vi "main_TC.vi"() -> ()   [LabVIEW 2017]
uses:
  <vilib>/addons/control/pid/pid.llb/PID (DBL).vi
  <vilib>/addons/control/pid/NI_PID_pid.lvlib
panel:
  out "Control_OnToOff":bool
  out "Abs Control Action":dbl
  in  "Tab Control":enum32{"Page 1", "Page 2"}(tab)
  in  "ON/OFF":bool
  in  "PID gains":cluster{"Kp":dbl, "KI":dbl, "Kd":dbl}={"Kp"=1.0, "KI"=0.0, "Kd"=0.0}
  in  "Pause Button":bool
  in  "Reset Chart":bool
  in  "Save as Excel":bool
  in  "Save as image":bool
  in  "Block Diagram":bool
  out "T3":dbl
  out "T2":dbl
  out "T1":dbl
  out "Cooler":bool
  out "Heater":bool
  out "Actuator Used":enum16{"heater", "cooler", "None"}(ring)
  out "Control Action":dbl
  in  "Temperature setpoint":dbl=25.0
  in  "Actuator":bool=TRUE
  in  "ON/OFF Control Loop":bool caption="ON/OFF control loop"
  in  "Exit":bool
  out "NI1":tag caption="NI device"
  out "Waveform Chart":T1(graph) caption="Response Chart"
  in  "Main board":bool
  # "Temperature Control Training System"
  # "Sensors Reading"
  # "Block Diagram of \nthe Temperature Closed-loop Control System"
  # "1"
  # "3"
  # "ON/OFF"
  # "ON/OFF Control Loop"
  # "Actuator ON/OFF"
  # "2"
  # "Heat Genration or \nAbsorption"
  # "Controller\n(PID)"
  # "Actuator\n(Heater/Cooler)"
  # "desired   T"
  # "Rod"
  # "error signal"
  # "+"
  # "-"
  # "Control Action\n(-100% - 100%)"
  # "T1"
  # "Sensors"
  # "T2"
  # "T3"
  # "Operation Steps :"
  # "1) Turn the Trainer switch ON\n2) Set the desired temperature \n3)Turn On the Control Loop switch\n\nNote: You can reset the desired temperature \n           while the control loop is running."
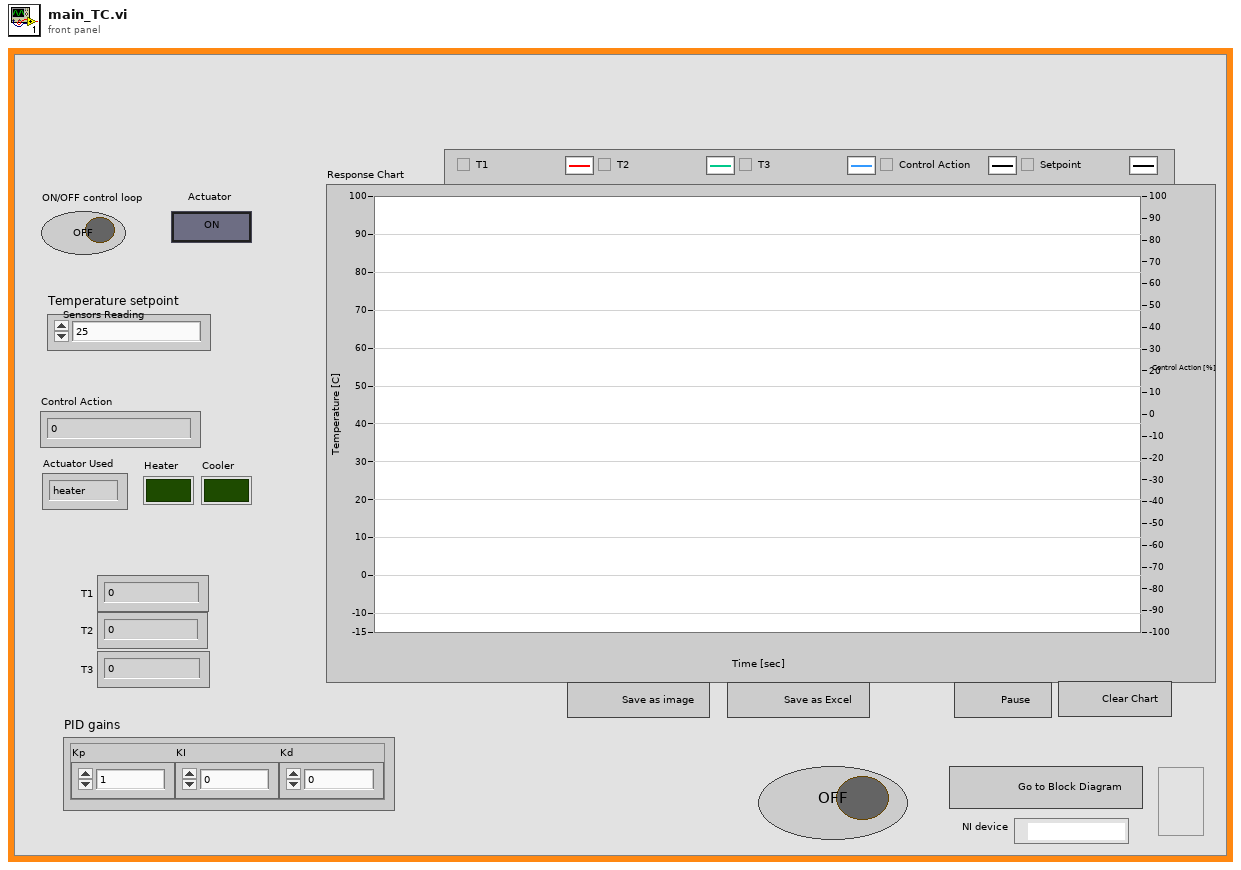
[diagram p1: front panel]
types:
  T1 = cluster{"Scalar":dbl, "Scalar":dbl, "Scalar":dbl, "f":dbl, "Temperature setpoint":dbl}
  T2 = enum32{"Invalid", "Standard", "Closed", "Hidden", "Minimized", "Maximized"}
  T3 = enum8{"Enabled", "Disabled", "Disabled and Grayed Out"}
  T4 = cluster{"Scalar":dbl, "Scalar":dbl, "Scalar":dbl, "f":dbl, "Temperature setpoint":dbl}[]
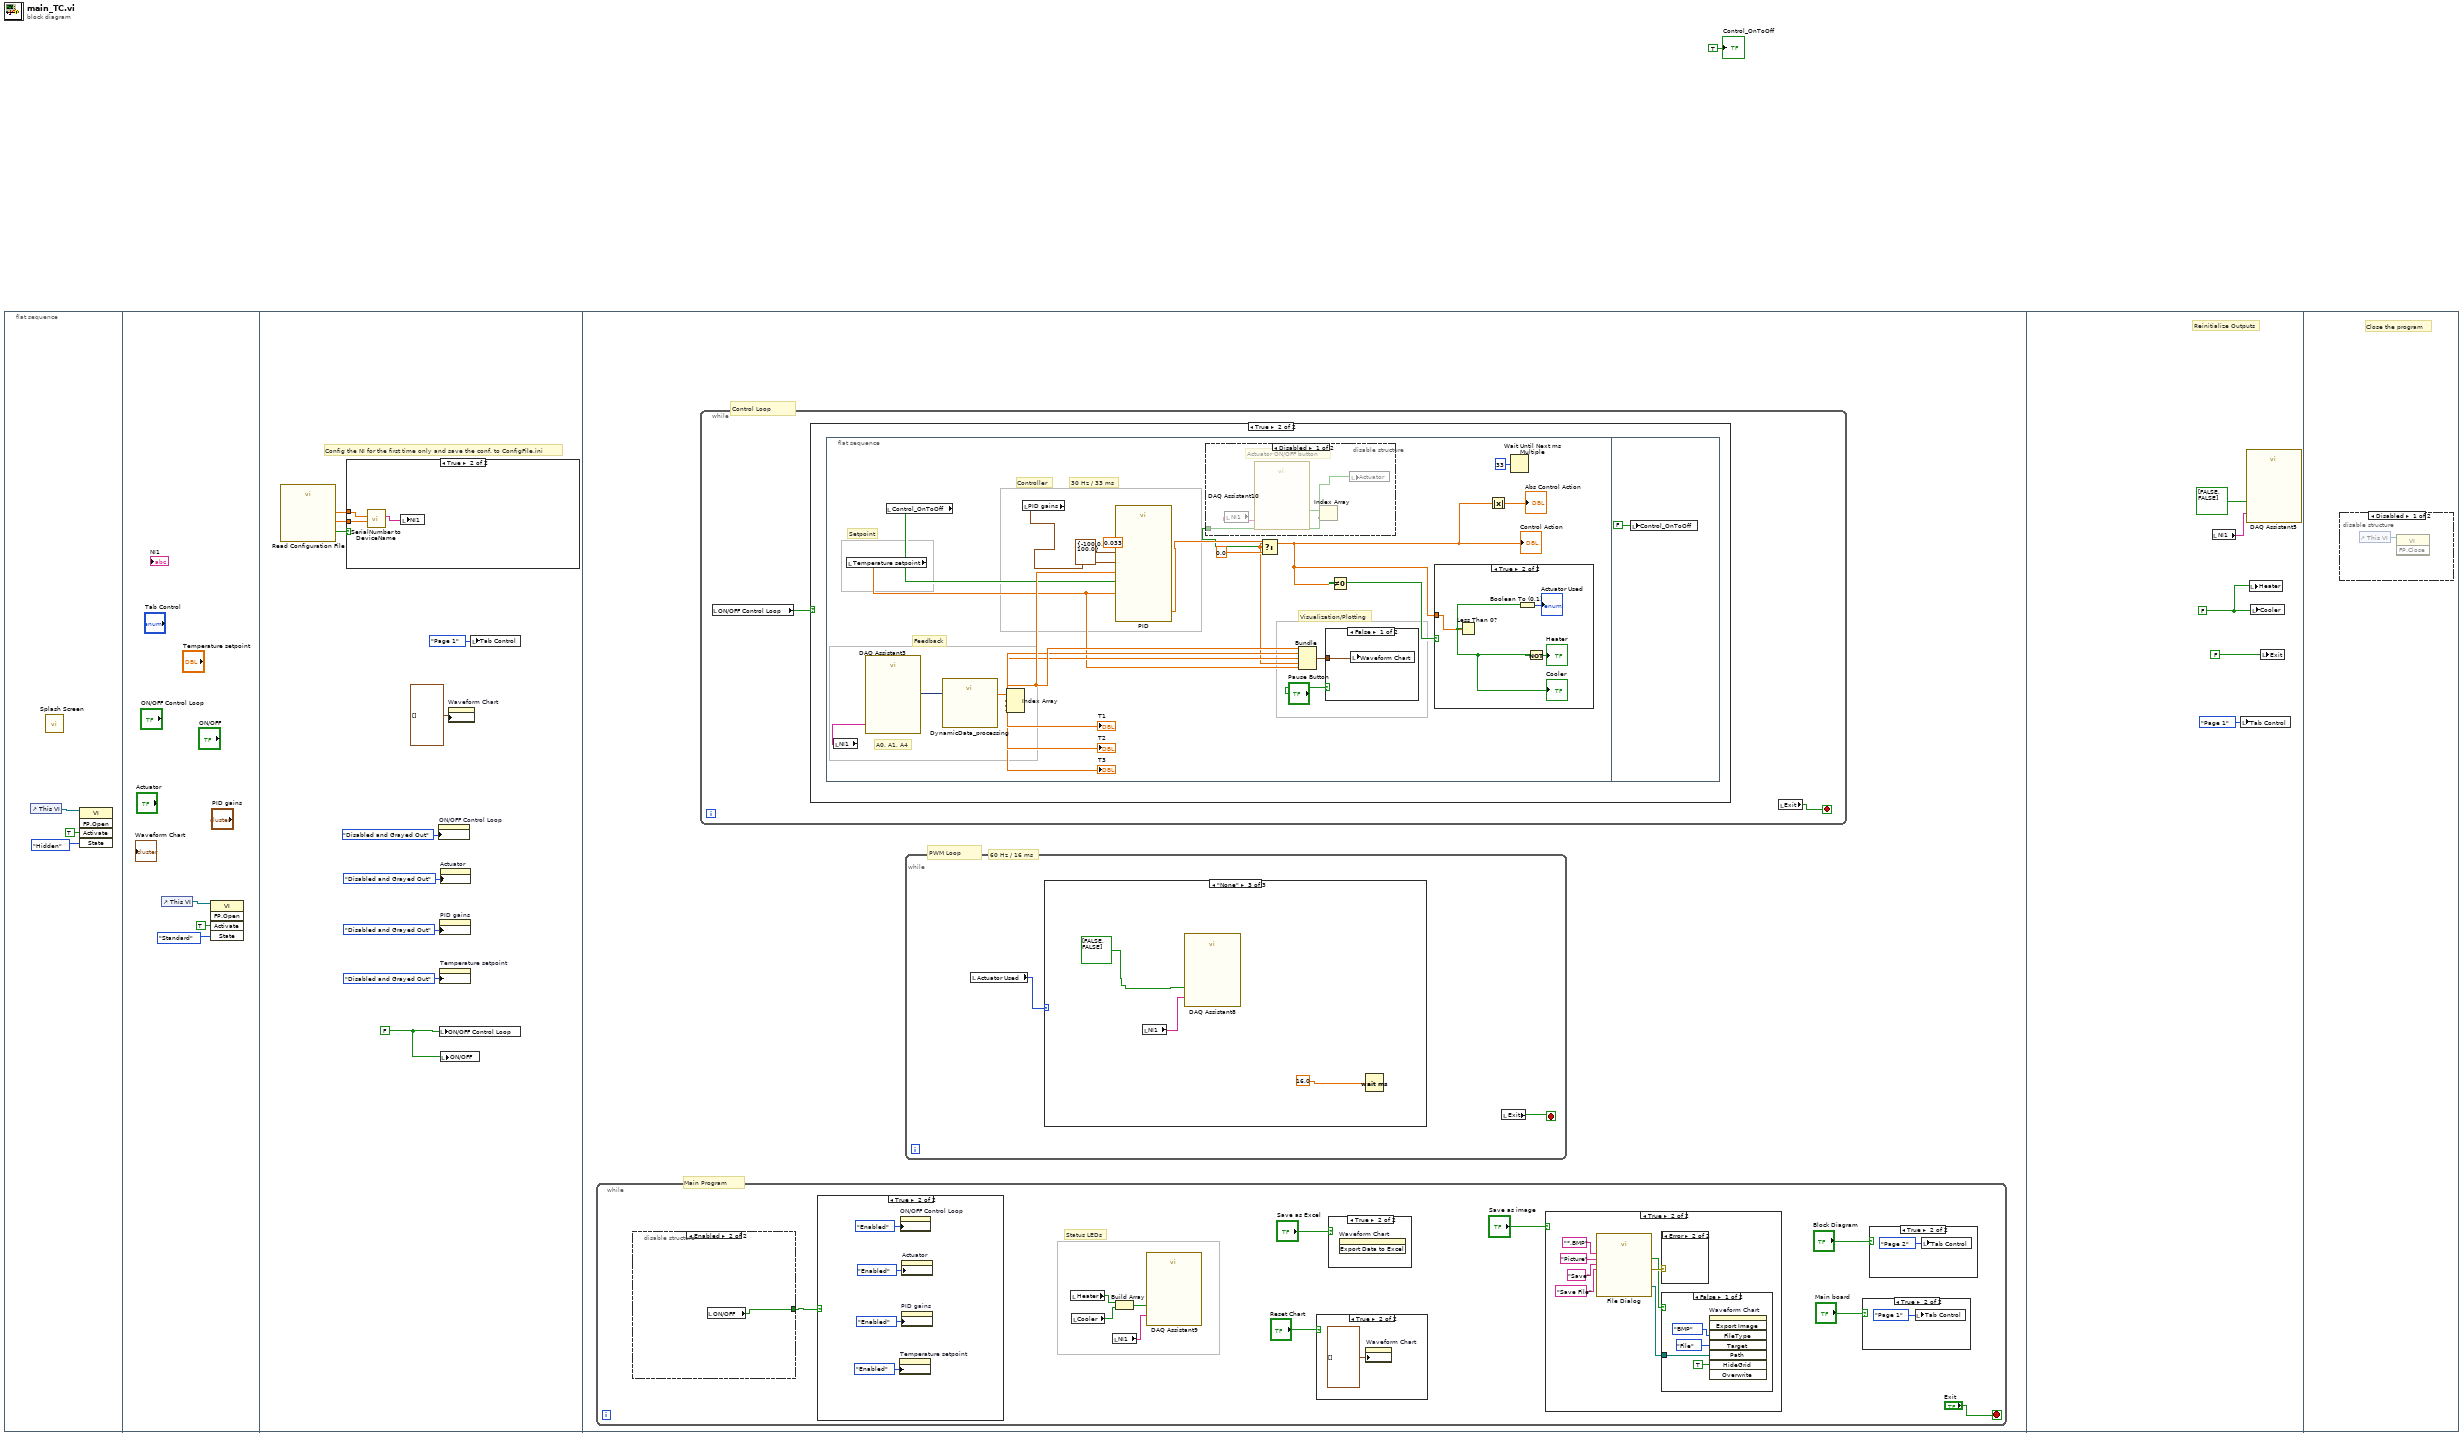
[diagram p0: block diagram]
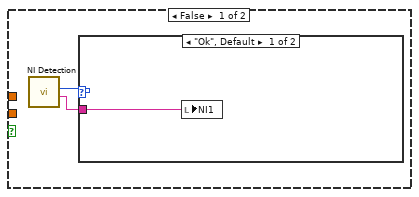
[diagram p2: hidden frame]
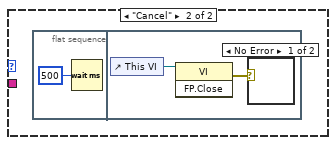
[diagram p3: hidden frame]
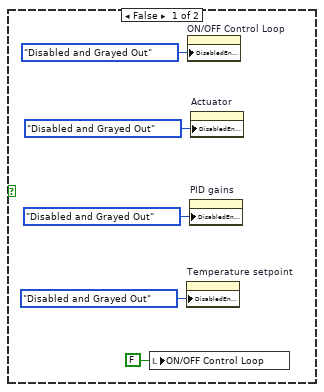
[diagram p5: hidden frame]
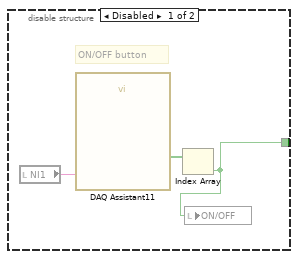
[diagram p6: hidden frame]
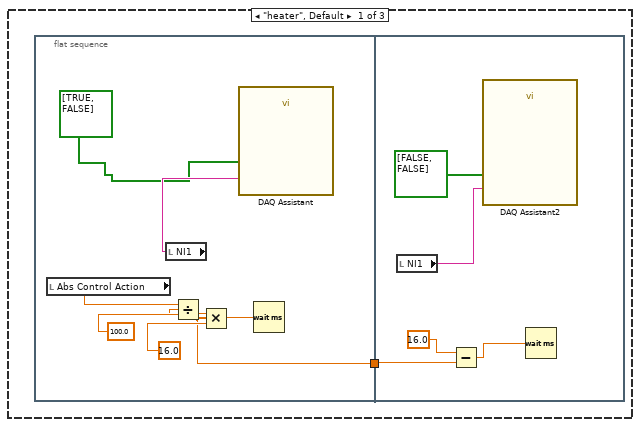
[diagram p14: hidden frame]
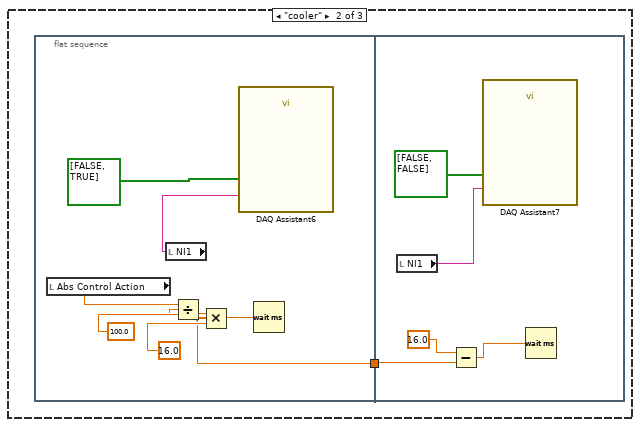
[diagram p15: hidden frame]
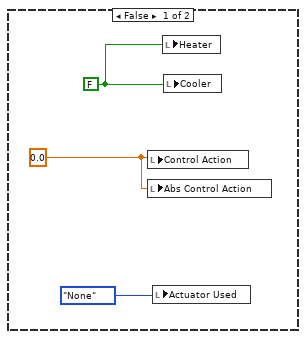
[diagram p16: hidden frame]
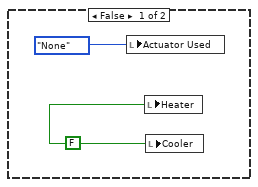
[diagram p18: hidden frame]
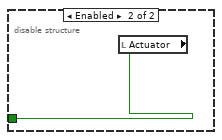
[diagram p19: hidden frame]
diagram:
  n1 = flat-sequence {
    frame #0 {
      n2 = control-ref of="This VI"() -> (w4:refnum<vi>)
      n3 = call "Splash Screen.vi"() -> ()  [unwired: 11 in, 1 out]
      n4 = invoke class="VI" method="FP.Open"(reference=w4, "Activate"=TRUE ("Activate?"), "State"=T2."Hidden") -> ()  [unwired: 2 in, 5 out]
    }
    frame #1 {
      n5 = control-ref of="This VI"() -> (w5:refnum<vi>)
      n6 = invoke class="VI" method="FP.Open"(reference=w5, "Activate"=TRUE ("Activate?"), "State"=T2."Standard") -> ()  [unwired: 2 in, 5 out]
    }
    frame #2 {
      w8 = FALSE ("ON/OFF Control Loop")
      # "Config the NI for the first time only and save the conf. to ConfigFile.ini"
      n7 = call "Read Configuration File.vi"() -> ("Serial Numbers Found"=w15:bool, "NI1"=w16:dbl, "NI2"=w17:dbl)  [unwired: 13 in]
      n8 = case shown="True" w15 {
        tunnel: w16 -> [_ w26]
        tunnel: w17 -> [_ w25]
        frame False {
          n9 = call "NI Detection.vi"() -> ("NI 1"=w18:tag, "Ok/Cancel"=w19:enum16{"Ok", "Cancel"})  [unwired: 8 in, 1 out]
          n10 = case shown="\"Ok\", Default" w19 {
            tunnel: w18 -> [w20 _]
            frame "Ok", Default {
              n11 = local write "NI1"(w20) -> ()
            }
            frame "Cancel" {
              n12 = flat-sequence {
                frame #0 {
                  n13 = Wait (ms)(milliseconds to wait=u32 500) -> ()  [unwired: 1 out]
                }
                frame #1 {
                  n14 = control-ref of="This VI"() -> (w23:refnum<vi>)
                  n15 = invoke class="VI" method="FP.Close"(reference=w23) -> (error out=w22:errorcluster)  [unwired: 2 in, 2 out]
                  n16 = case shown="No Error" w22 {
                    frame No Error {
                    }
                    frame Error {
                    }
                  }
                }
              }
            }
          }
        }
        frame True {
          n17 = call "SerialNumber to DeviceName.vi"("NI2 Serial Number"=w25, "NI1 Serial Number"=w26) -> ("NI1 Device Name"=w24:tag)  [unwired: 8 in, 1 out]
          n18 = local write "NI1"(w24) -> ()
        }
      }
      n19 = property on="ON/OFF Control Loop" class="Bool (strict)"("DisabledEnum"=T3."Disabled and Grayed Out" ("Disabled")) -> ()  [unwired: 2 in, 2 out]
      n20 = local write "ON/OFF Control Loop"(w8) -> ()
      n21 = property on="PID gains" class="Clust (strict)"("DisabledEnum"=T3."Disabled and Grayed Out" ("Disabled")) -> ()  [unwired: 2 in, 2 out]
      n22 = property on="Temperature setpoint" class="DigNum (strict)"("DisabledEnum"=T3."Disabled and Grayed Out" ("Disabled")) -> ()  [unwired: 2 in, 2 out]
      n23 = property on="Actuator" class="Bool (strict)"("DisabledEnum"=T3."Disabled and Grayed Out" ("Disabled")) -> ()  [unwired: 2 in, 2 out]
      n24 = local write "ON/OFF"(w8) -> ()
      n25 = property on="Waveform Chart" class="WFChart (strict)"("History Data"=T4 []) -> ()  [unwired: 2 in, 2 out]
      n26 = local write "Tab Control"(enum32{"Page 1", "Page 2"}."Page 1" ("Tab Control")) -> ()
    }
    frame #3 {
      # "Main Program"
      # "60 Hz / 16 ms"
      # "PWM Loop"
      # "Control Loop"
      n27 = while {
        stop <- "Exit" stop-if-true
        # "Status LEDs"
        n28 = disable-structure shown="Enabled" {
          disable-tunnel: [w47 w50] -> w28
          frame Disabled {
            # "ON/OFF button"
            n29 = local read "NI1"() -> (w49:tag)
            n30 = call "DAQ Assistant11"("device name"=w49) -> ("data"=w48:bool[])  [unwired: 16 in, 2 out]
            n31 = Index Array(array=w48) -> (element=w47:bool)  [unwired: 1 in]
            n32 = local write "ON/OFF"(w47) -> ()
          }
          frame Enabled {
            n33 = local read "ON/OFF"() -> (w50:bool)
          }
        }
        n34 = case shown="True" w28 {
          frame False {
            n35 = local write "ON/OFF Control Loop"(FALSE ("ON/OFF Control Loop")) -> ()
            n36 = property on="Temperature setpoint" class="DigNum (strict)"("DisabledEnum"=T3."Disabled and Grayed Out" ("Disabled")) -> ()  [unwired: 2 in, 2 out]
            n37 = property on="ON/OFF Control Loop" class="Bool (strict)"("DisabledEnum"=T3."Disabled and Grayed Out" ("Disabled")) -> ()  [unwired: 2 in, 2 out]
            n38 = property on="PID gains" class="Clust (strict)"("DisabledEnum"=T3."Disabled and Grayed Out" ("Disabled")) -> ()  [unwired: 2 in, 2 out]
            n39 = property on="Actuator" class="Bool (strict)"("DisabledEnum"=T3."Disabled and Grayed Out" ("Disabled")) -> ()  [unwired: 2 in, 2 out]
          }
          frame True {
            n40 = property on="Temperature setpoint" class="DigNum (strict)"("DisabledEnum"=T3."Enabled" ("Disabled")) -> ()  [unwired: 2 in, 2 out]
            n41 = property on="ON/OFF Control Loop" class="Bool (strict)"("DisabledEnum"=T3."Enabled" ("Disabled")) -> ()  [unwired: 2 in, 2 out]
            n42 = property on="PID gains" class="Clust (strict)"("DisabledEnum"=T3."Enabled" ("Disabled")) -> ()  [unwired: 2 in, 2 out]
            n43 = property on="Actuator" class="Bool (strict)"("DisabledEnum"=T3."Enabled" ("Disabled")) -> ()  [unwired: 2 in, 2 out]
          }
        }
        n44 = local read "Heater"() -> (w32:bool)
        n45 = local read "Cooler"() -> (w31:bool)
        n46 = local read "NI1"() -> (w29:tag)
        n47 = Build Array(w32, w31) -> (w30:bool[])
        n48 = call "DAQ Assistant9"("data"=w30, "device name"=w29) -> ()  [unwired: 16 in, 2 out]
        n49 = case shown="True" "Reset Chart" {
          frame False {
          }
          frame True {
            n50 = property on="Waveform Chart" class="WFChart (strict)"("History Data"=T4 []) -> ()  [unwired: 2 in, 2 out]
          }
        }
        n51 = case shown="True" "Save as Excel" {
          frame False {
          }
          frame True {
            n52 = invoke on="Waveform Chart" class="WFChart (strict)" method="Export Data to Excel"() -> ()  [unwired: 3 in, 3 out]
          }
        }
        n53 = case shown="True" "Save as image" {
          frame False {
          }
          frame True {
            n54 = call "File Dialog"("prompt"="Save File", "button label"="Save", "pattern (all files)"="*.BMP", "pattern label"="Picture") -> ("selected path"=w52:path, "cancelled"=w51:bool, "error out"=w53:errorcluster)  [unwired: 8 in, 1 out]
            n55 = case shown="Error" w53 {
              frame No Error {
              }
              frame Error {
              }
            }
            n56 = case shown="False" w51 {
              tunnel: w52 -> [w59 _]
              frame False {
                n57 = invoke on="Waveform Chart" class="WFChart (strict)" method="Export Image"("FileType"=enum32{"BMP", "EPS", "EMF", "PICT"}."BMP" ("File Type"), "Target"=enum32{"File", "Clipboard"}."File", "Path"=w59, "HideGrid"=TRUE ("Hide Grid")) -> ()  [unwired: 4 in, 8 out]
              }
              frame True {
              }
            }
          }
        }
        n58 = case shown="True" "Main board" {
          frame False {
          }
          frame True {
            n59 = local write "Tab Control"(enum32{"Page 1", "Page 2"}."Page 1" ("Tab Control")) -> ()
          }
        }
        n60 = case shown="True" "Block Diagram" {
          frame False {
          }
          frame True {
            n61 = local write "Tab Control"(enum32{"Page 1", "Page 2"}."Page 2" ("Tab Control")) -> ()
          }
        }
      }
      n62 = while {
        stop <- w96 stop-if-true
        n63 = local read "ON/OFF Control Loop"() -> (w97:bool)
        n64 = case shown="True" w97 {
          frame False {
            w100 = 0.0 ("Control Action")
            w99 = FALSE ("Heater")
            n65 = local write "Control Action"(w100) -> ()
            n66 = local write "Abs Control Action"(w100) -> ()
            n67 = local write "Actuator Used"(enum16{"heater", "cooler", "None"}."None" ("Actuator Used 2")) -> ()
            n68 = local write "Heater"(w99) -> ()
            n69 = local write "Cooler"(w99) -> ()
          }
          frame True {
            n70 = flat-sequence {
              frame #0 {
                # "Setpoint"
                # "Visualization/Plotting"
                # "Controller"
                # "Feedback"
                # "30 Hz / 33 ms"
                # "A0, A1, A4"
                n71 = local read "NI1"() -> (w110:tag)
                n72 = local read "Temperature setpoint"() -> (w102:dbl)
                n73 = call "DAQ Assistant3"("device name"=w110) -> ("data"=w120:dynamicdata)  [unwired: 16 in, 2 out]
                n74 = local read "Control_OnToOff"() -> (w101:bool)
                n75 = call "DynamicData_processing.vi"("data"=w120) -> ("DATA"=w119:dbl[])
                n76 = Index Array(array=w119) -> (element #1=w114:dbl, element #2=w113:dbl, element #3=w112:dbl)  [unwired: 3 in]
                "T1" <- w114
                "T2" <- w113
                "T3" <- w112
                n77 = local read "PID gains"() -> (w103:cluster{"Kp":dbl, "KI":dbl, "Kd":dbl})
                n78 = call-poly <vilib>:"PID.vi"("reinitialize? (F)"=w101, "output range"=cluster{"output high":dbl, "output low":dbl} {"output high"=-100.0, "output low"=100.0}, "dt (s)"=0.033, "PID gains"=w103, "process variable"=w114, "setpoint"=w102) -> ("output"=w117:dbl)  [unwired: 4 in, 1 out]
                n79 = disable-structure shown="Disabled" {
                  disable-tunnel: [w129 w131] -> w104
                  frame Disabled {
                    # "Actuator ON/OFF button"
                    n80 = local read "NI1"() -> (w128:tag)
                    n81 = call "DAQ Assistant10"("device name"=w128) -> ("data"=w130:bool[])  [unwired: 16 in, 2 out]
                    n82 = Index Array(array=w130) -> (element=w129:bool)  [unwired: 1 in]
                    n83 = local write "Actuator"(w129) -> ()
                  }
                  frame Enabled {
                    n84 = local read "Actuator"() -> (w131:bool)
                  }
                }
                n85 = Select(t=w117, s=w104, f=0.0) -> (s? t:f=w106:dbl)
                "Control Action" <- w106
                n86 = Bundle("Scalar"=w114, "Scalar"=w113, "Scalar"=w112, "f"=w106, "Temperature setpoint"=w102) -> (w111:T1)  [unwired: 1 in]
                n87 = case shown="False" "Pause Button" {
                  tunnel: w111 -> [w121 _]
                  frame False {
                    n88 = local write "Waveform Chart"(w121) -> ()
                  }
                  frame True {
                  }
                }
                n89 = Not Equal To 0?(x=w106) -> (x != 0?=w107:bool)
                n90 = case shown="True" w107 {
                  tunnel: w106 -> [_ w125]
                  frame False {
                    w122 = FALSE ("Heater")
                    n91 = local write "Actuator Used"(enum16{"heater", "cooler", "None"}."None" ("Actuator Used 2")) -> ()
                    n92 = local write "Heater"(w122) -> ()
                    n93 = local write "Cooler"(w122) -> ()
                  }
                  frame True {
                    n94 = Less Than 0?(x=w125) -> (x < 0?=w124:bool)
                    "Cooler" <- w124
                    n95 = Boolean To (0,1)(Boolean=w124) -> (0, 1=→"Actuator Used":i16)
                    n96 = Not(x=w124) -> (.not. x?=→"Heater":bool)
                  }
                }
                n97 = Absolute Value(x=w106) -> (abs(x)=→"Abs Control Action":dbl)
                n98 = Wait Until Next ms Multiple(millisecond multiple=u32 33) -> ()  [unwired: 1 out]
              }
              frame #1 {
                n99 = local write "Control_OnToOff"(FALSE ("Control_OnToOff")) -> ()
              }
            }
          }
        }
        n100 = local read "Exit"() -> (w96:bool)
      }
      n101 = while {
        stop <- w65 stop-if-true
        n102 = local read "Actuator Used"() -> (w66:enum16{"heater", "cooler", "None"})
        n103 = case shown="\"None\"" w66 {
          frame "heater", Default {
            n104 = flat-sequence {
              tunnel: [w71] -> w67
              tunnel: w67 -> [w79]
              frame #0 {
                n105 = local read "Abs Control Action"() -> (w69:dbl)
                n106 = local read "NI1"() -> (w70:tag)
                n107 = Divide(x=w69, y=100.0) -> (x/y=w73:dbl)
                n108 = Multiply(x=w73, y=16.0) -> (x*y=w71:dbl)
                n109 = call "DAQ Assistant"("data"=bool[] [TRUE, FALSE], "device name"=w70) -> ()  [unwired: 16 in, 2 out]
                n110 = Wait (ms)(milliseconds to wait=w71) -> ()  [unwired: 1 out]
              }
              frame #1 {
                n111 = local read "NI1"() -> (w76:tag)
                n112 = Subtract(x=16.0 ("y"), y=w79) -> (x-y=w77:dbl)
                n113 = call "DAQ Assistant2"("data"=bool[] [FALSE, FALSE], "device name"=w76) -> ()  [unwired: 16 in, 2 out]
                n114 = Wait (ms)(milliseconds to wait=w77) -> ()  [unwired: 1 out]
              }
            }
          }
          frame "cooler" {
            n115 = flat-sequence {
              tunnel: [w84] -> w80
              tunnel: w80 -> [w92]
              frame #0 {
                n116 = local read "Abs Control Action"() -> (w82:dbl)
                n117 = local read "NI1"() -> (w83:tag)
                n118 = Divide(x=w82, y=100.0) -> (x/y=w86:dbl)
                n119 = Multiply(x=w86, y=16.0) -> (x*y=w84:dbl)
                n120 = call "DAQ Assistant6"("data"=bool[] [FALSE, TRUE], "device name"=w83) -> ()  [unwired: 16 in, 2 out]
                n121 = Wait (ms)(milliseconds to wait=w84) -> ()  [unwired: 1 out]
              }
              frame #1 {
                n122 = local read "NI1"() -> (w89:tag)
                n123 = Subtract(x=16.0 ("y"), y=w92) -> (x-y=w90:dbl)
                n124 = call "DAQ Assistant7"("data"=bool[] [FALSE, FALSE], "device name"=w89) -> ()  [unwired: 16 in, 2 out]
                n125 = Wait (ms)(milliseconds to wait=w90) -> ()  [unwired: 1 out]
              }
            }
          }
          frame "None" {
            n126 = local read "NI1"() -> (w95:tag)
            n127 = call "DAQ Assistant8"("data"=bool[] [FALSE, FALSE], "device name"=w95) -> ()  [unwired: 16 in, 2 out]
            n128 = Wait (ms)(milliseconds to wait=16.0 ("y")) -> ()  [unwired: 1 out]
          }
        }
        n129 = local read "Exit"() -> (w65:bool)
      }
    }
    frame #4 {
      w135 = FALSE ("Heater")
      # "Reinitialize Outputs"
      n130 = local read "NI1"() -> (w136:tag)
      n131 = local write "Tab Control"(enum32{"Page 1", "Page 2"}."Page 1" ("Tab Control")) -> ()
      n132 = call "DAQ Assistant5"("data"=bool[] [FALSE, FALSE], "device name"=w136) -> ()  [unwired: 16 in, 2 out]
      n133 = local write "Heater"(w135) -> ()
      n134 = local write "Cooler"(w135) -> ()
      n135 = local write "Exit"(FALSE ("Exit")) -> ()
    }
    frame #5 {
      # "Close the program"
      n136 = disable-structure shown="Disabled" {
        frame Disabled {
          n137 = control-ref of="This VI"() -> (w138:refnum<vi>)
          n138 = invoke class="VI" method="FP.Close"(reference=w138) -> ()  [unwired: 2 in, 3 out]
        }
        frame Enabled {
        }
      }
    }
  }
  "Control_OnToOff" <- TRUE ("Boolean")
